vi "Main.vi"() -> ()   [LabVIEW 2018]
uses:
  FGV/FGV_mods.ctl
panel:
  out "graph":cluster{"X":u32[], "Y":u32[]}[](graph) caption="XY Graph"
  in  "file":path caption="Arquivo"
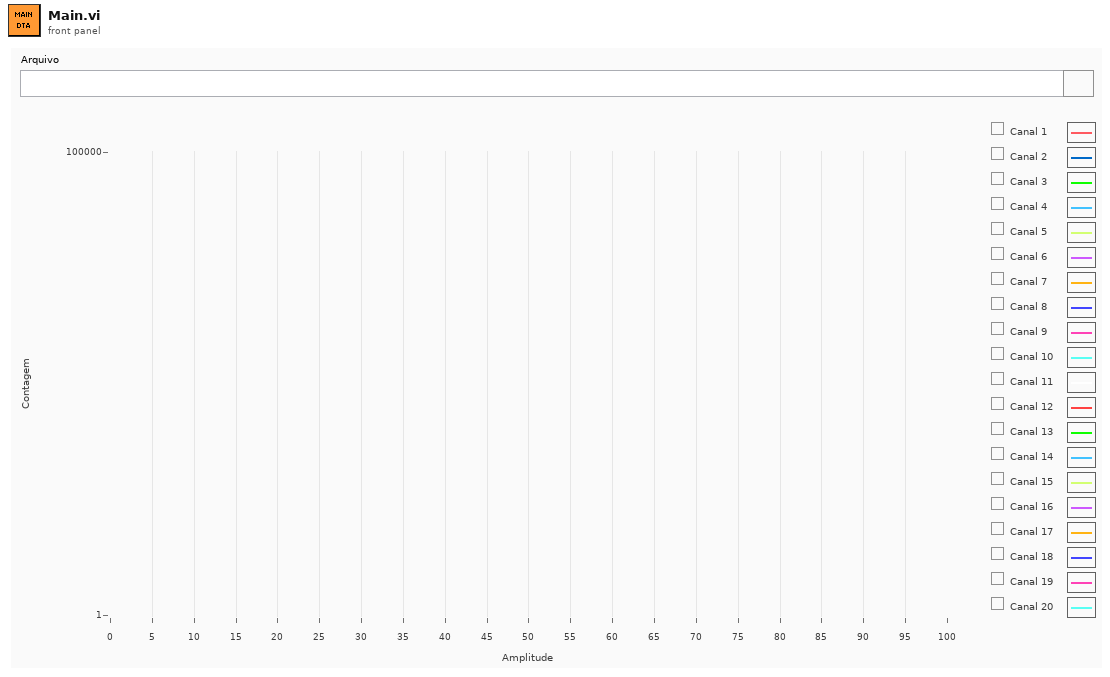
[diagram p1: front panel]
types:
  T1 = typedef "FGV_mods.ctl" = enum16{"Init", "get_config", "get_hits", "set_file", "open_file", "close"}
  T2 = typedef "hit_data.ctl" = cluster{"channel":u8, "time":dbl, "parameters":cluster{"riseTime":u32, "countsToPeak":u32, "counts":u32, "energy":u32, "duration":u32, "amplitude":u32, "RMS":u32, "ASL":u32, "gain":u32, "THR":u32, "preAmp":u32, "avrFreq":u32}}
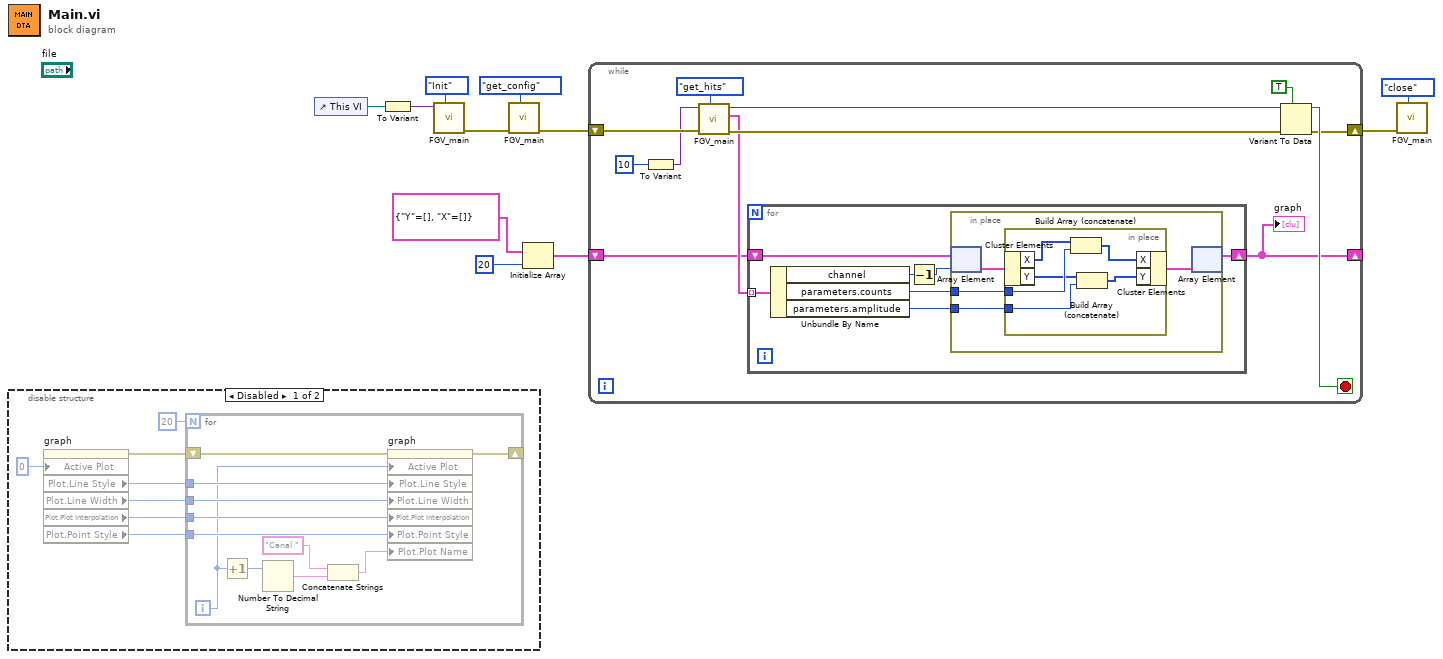
[diagram p0: block diagram]
diagram:
  n1 = disable-structure shown="Disabled" {
    frame Disabled {
      n2 = property on="graph" class="XYGraph (strict)"("Active Plot"=u32 0) -> (error out=w17:errorcluster, "Plot.Line Style"=w15:u8, "Plot.Line Width"=w14:u8, "Plot.Plot Interpolation"=w13:u8, "Plot.Point Style"=w12:u8)  [unwired: 2 in, 1 out]
      n3 = for {
        N: 20 -> [_]
        shift-right: [w28] -> _
        shift-left: w17 -> [w29]
        tunnel: w15 -> [w27]
        tunnel: w14 -> [w26]
        tunnel: w13 -> [w25]
        tunnel: w12 -> [w24]
        i -> [w23]
        n4 = Increment(x=w23) -> (x+1=w19:i32)
        n5 = Number To Decimal String(number=w19) -> (decimal integer string=w22:string)  [unwired: 1 in]
        n6 = Concatenate Strings("Canal " ("string"), w22) -> (w20:string)
        n7 = property on="graph" class="XYGraph (strict)"(error in=w29, "Active Plot"=w23, "Plot.Line Style"=w27, "Plot.Line Width"=w26, "Plot.Plot Interpolation"=w25, "Plot.Point Style"=w24, "Plot.Plot Name"=w20) -> (error out=w28:errorcluster)  [unwired: 1 in, 1 out]
      }
    }
    frame Enabled {
    }
  }
  n8 = control-ref of="This VI"() -> (w2:refnum<vi>)
  n9 = To Variant(anything=w2) -> (Variant=w1:variant)
  n10 = call "FGV_main.vi"("FGV_mods"=FGV_mods."Init", "DataIn"=w1) -> ("Error Out"=w9:errorcluster)  [unwired: 7 in, 2 out]
  n11 = call "FGV_main.vi"("FGV_mods"=FGV_mods."get_config", "Error In"=w9) -> ("Error Out"=w8:errorcluster)  [unwired: 7 in, 2 out]
  n12 = Initialize Array(cluster{"Y":u32[], "X":u32[]} {"Y"=[], "X"=[]}, 20 ("dimension size")) -> (w3:cluster{"Y":u32[], "X":u32[]}[])
  n13 = while {
    shift-right: [w33] -> w6
    shift-left: w8 -> [w40]
    shift-right: [w30] -> _
    shift-left: w3 -> [w31]
    stop <- w35 stop-if-true
    n14 = To Variant(anything=10) -> (Variant=w38:variant)
    n15 = call "FGV_main.vi"("FGV_mods"=FGV_mods."get_hits", "Error In"=w40, "DataIn"=w38) -> ("Error Out"=w34:errorcluster, "hits"=w32:T2[], "DataOut"=w37:variant)  [unwired: 6 in]
    n16 = for {
      tunnel: w32 -> [w47] mode=indexing
      shift-right: [w43] -> w30
      shift-left: w31 -> [w48]
      n17 = Unbundle By Name(w47) -> ("channel"=w46:u8, "parameters.counts"=w45:u32, "parameters.amplitude"=w44:u32)
      n18 = Decrement(x=w46) -> (x-1=w42:u8)
      n19 = in-place {
        in-place-border: w45 -> [w51]
        in-place-border: w44 -> [w50]
        n20 = in-place-array #1(w48, w42) -> (w52:cluster{"Y":u32[], "X":u32[]})
        n21 = in-place {
          in-place-border: w51 -> [w57]
          in-place-border: w50 -> [w54]
          n22 = in-place-cluster #2(w52) -> ("X"=w58:u32[], "Y"=w55:u32[])
          n23 = Build Array (concatenate)(w58, w57) -> (w56:u32[])
          n24 = Build Array (concatenate)(w55, w54) -> (w53:u32[])
          n25 = in-place-cluster #2("X"=w56, "Y"=w53) -> (w49:cluster{"Y":u32[], "X":u32[]})
        }
        n26 = in-place-array #1(w49) -> (w43:cluster{"Y":u32[], "X":u32[]}[])  [unwired: 1 out]
      }
    }
    "graph" <- w30
    n27 = Variant To Data(error in=w34, type=TRUE, Variant=w37) -> (data=w35:bool, error out=w33:errorcluster)
  }
  n28 = call "FGV_main.vi"("FGV_mods"=FGV_mods."close", "Error In"=w6) -> ()  [unwired: 7 in, 3 out]
